vi "Parse Parameters File.vi"(8 "error in":errorcluster, 11 "path to XML document":path caption="path to parameters xml") -> (0 "error out":errorcluster, 2 "board configuration out":T1 {"portConfiguration"."Rx_UDP"."Tx_UDP"."FilterMode" items=["FDX_RX_VL_FLT_DIS", "FDX_RX_VL_FLT_ENA ", "FDX_RX_VL_FLT_ENA_INV"]; "portConfiguration"."Rx_UDP"."Tx_UDP"."VLBufSize" format="%.0x"; "portConfiguration"."Rx_UDP"."Tx_UDP"."VerificationMode" items=["FDX_RX_VL_CHECK_ENA_DEFAULT"=65535, "FDX_RX_VL_CHECK_REDMAM"=16, "DX_RX_VL_CHECK_TRAFIC"=8, "FDX_RX_VL_CHECK_FRAMESIZE"=4, "FDX_RX_VL_CHECK_SNINTEG"=2, "FDX_RX_VL_CHECK_INVPAC"=1, "FDX_RX_VL_CHECK_DISA"=0]; "portConfiguration"."Tx_UDP"."tx_udp_setup"."interfaceID" format="%.0b"; "portConfiguration"."Tx_UDP"."tx_udp_setup"."NetSelect" items=["FDX_TX_FRAME_DLY_A"=0, "FDX_TX_FRAME_DLY_B"=1, "FDX_TX_FRAME_BOTH "=3, "FDX_TX_FRAME_ONLY_A"=4, "FDX_TX_FRAME_ONLY_B "=5]; "portConfiguration"."Rx_Monitor"."Strobe" items=["FDX_MON_STROBE_DIS", "FDX_MON_STROBE_STOP", "FDX_MON_STROBE_START"]; "portConfiguration"."Rx_Monitor"."CaptureMode" items=["FDX_MON_SINGLE ", "FDX_MON_CONTINUOUS", "FDX_MON_SELECTIVE", "FDX_MON_RECORDING", "FDX_MON_REROS", "FDX_MON_HMU"]; "portConfiguration"."Rx_Monitor"."DefaultCronoMode" items=["FDX_RX_DEFAULT_ENA_CNT", "FDX_RX_DEFAULT_MON_ENA_ALL", "FDX_RX_DEFAULT_MON_ENA_GOOD"]; "portConfiguration"."Tx_Generic"."Frame Headers"."Frame header"."PhysErrorInjection" items=["FDX_TX_FRAME_ERR_OFF", "FDX_TX_FRAME_ERR_CRC", "FDX_TX_FRAME_ERR_ALI", "FDX_TX_FRAME_ERR_PRE", "FDX_TX_FRAME_ERR_PHY"]; "portConfiguration"."Tx_Generic"."Frame Headers"."Frame header"."PayloadGenerationMode" items=["FDX_TX_FRAME_PGM_USER", "FDX_TX_FRAME_PGM_IP_PART", "FDX_TX_FRAME_PGM_IP_PART_TT", "FDX_TX_FRAME_PGM_IP_FULL", "FDX_TX_FRAME_PGM_IP_FULL_TT"]; "portConfiguration"."Tx_Generic"."Frame Headers"."Frame header"."PayloadBufferMode" items=["FDX_TX_FRAME_PBM_STD", "FDX_TX_FRAME_PBM_MAC", "FDX_TX_FRAME_PBM_UDP", "FDX_TX_FRAME_PBM_FULL"]; "portConfiguration"."Tx_Generic"."Frame Headers"."Frame header"."NetSelect" items=["FDX_TX_FRAME_DLY_A"=0, "FDX_TX_FRAME_DLY_B"=1, "FDX_TX_FRAME_BOTH "=3, "FDX_TX_FRAME_ONLY_A"=4, "FDX_TX_FRAME_ONLY_B "=5]; "portConfiguration"."Tx_Generic"."Frame Headers"."Frame header"."FrameStartMode" items=["FDX_TX_FRAME_START_IFG", "FDX_TX_FRAME_START_PGWT", "FDX_TX_FRAME_START_TRG", "FDX_TX_FRAME_START_TRG_D"]; "portConfiguration"."Tx_Generic"."tx_generic_setup"."StartMode" items=["FDX_STOP", "FDX_START", "FDX_START_TRG", "FDX_START_TIME"]; "boardSetup"."portConfig" items=["FDX_SINGLE", "FDX_REDUNDANT"]; "boardSetup"."portSpeed" items=["FDX_100MBIT", "FDX_10MBIT", "FDX_AUTO_100MBIT", "FDX_AUTO_10MBIT", "FDX_AUTO_ERROR", "FDX_1000MBIT"]}, 3 "path to XML document out":path caption="path to parameters xml")   [LabVIEW 2020, in "AIM ARINC 664 Import.lvlib"]
uses:
  AIM ARINC 664 Import.lvlib
  <vilib>/xml/NI_XML.lvlib
  <resource>/objmgr/DOMUserDefRef.rc
  _typedefs/Board Top Level Configuration.ctl
  _typedefs/board_setup.ctl
  _typedefs/port_tx_udp_sap.ctl
  _typedefs/port_tx_udp_comm.ctl
  _typedefs/tx_udp_setup.ctl
  _typedefs/port_setup.ctl
  _typedefs/port_configuration.ctl
  _typedefs/port_rx_udp_sap.ctl
  _typedefs/port_rx_udp_comm.ctl
  _typedefs/rx_udp_setup.ctl
  _typedefs/frame_parameter.ctl
  _typedefs/frame_parameter_definition.ctl
  _typedefs/session_tx_generic.ctl
  _typedefs/frame_tx_generic_seqNumberOffset.ctl
  _typedefs/frame_tx_generic_seqNumberInit.ctl
  _typedefs/tx_generic_setup.ctl
  _typedefs/session_rx_monitor.ctl
  <vilib>/xml/Load XML File.vi
  _typedefs/frame_tx_generic.ctl
  Shared/Encoding (Arinc664).ctl
panel:
  out "parse errors":string
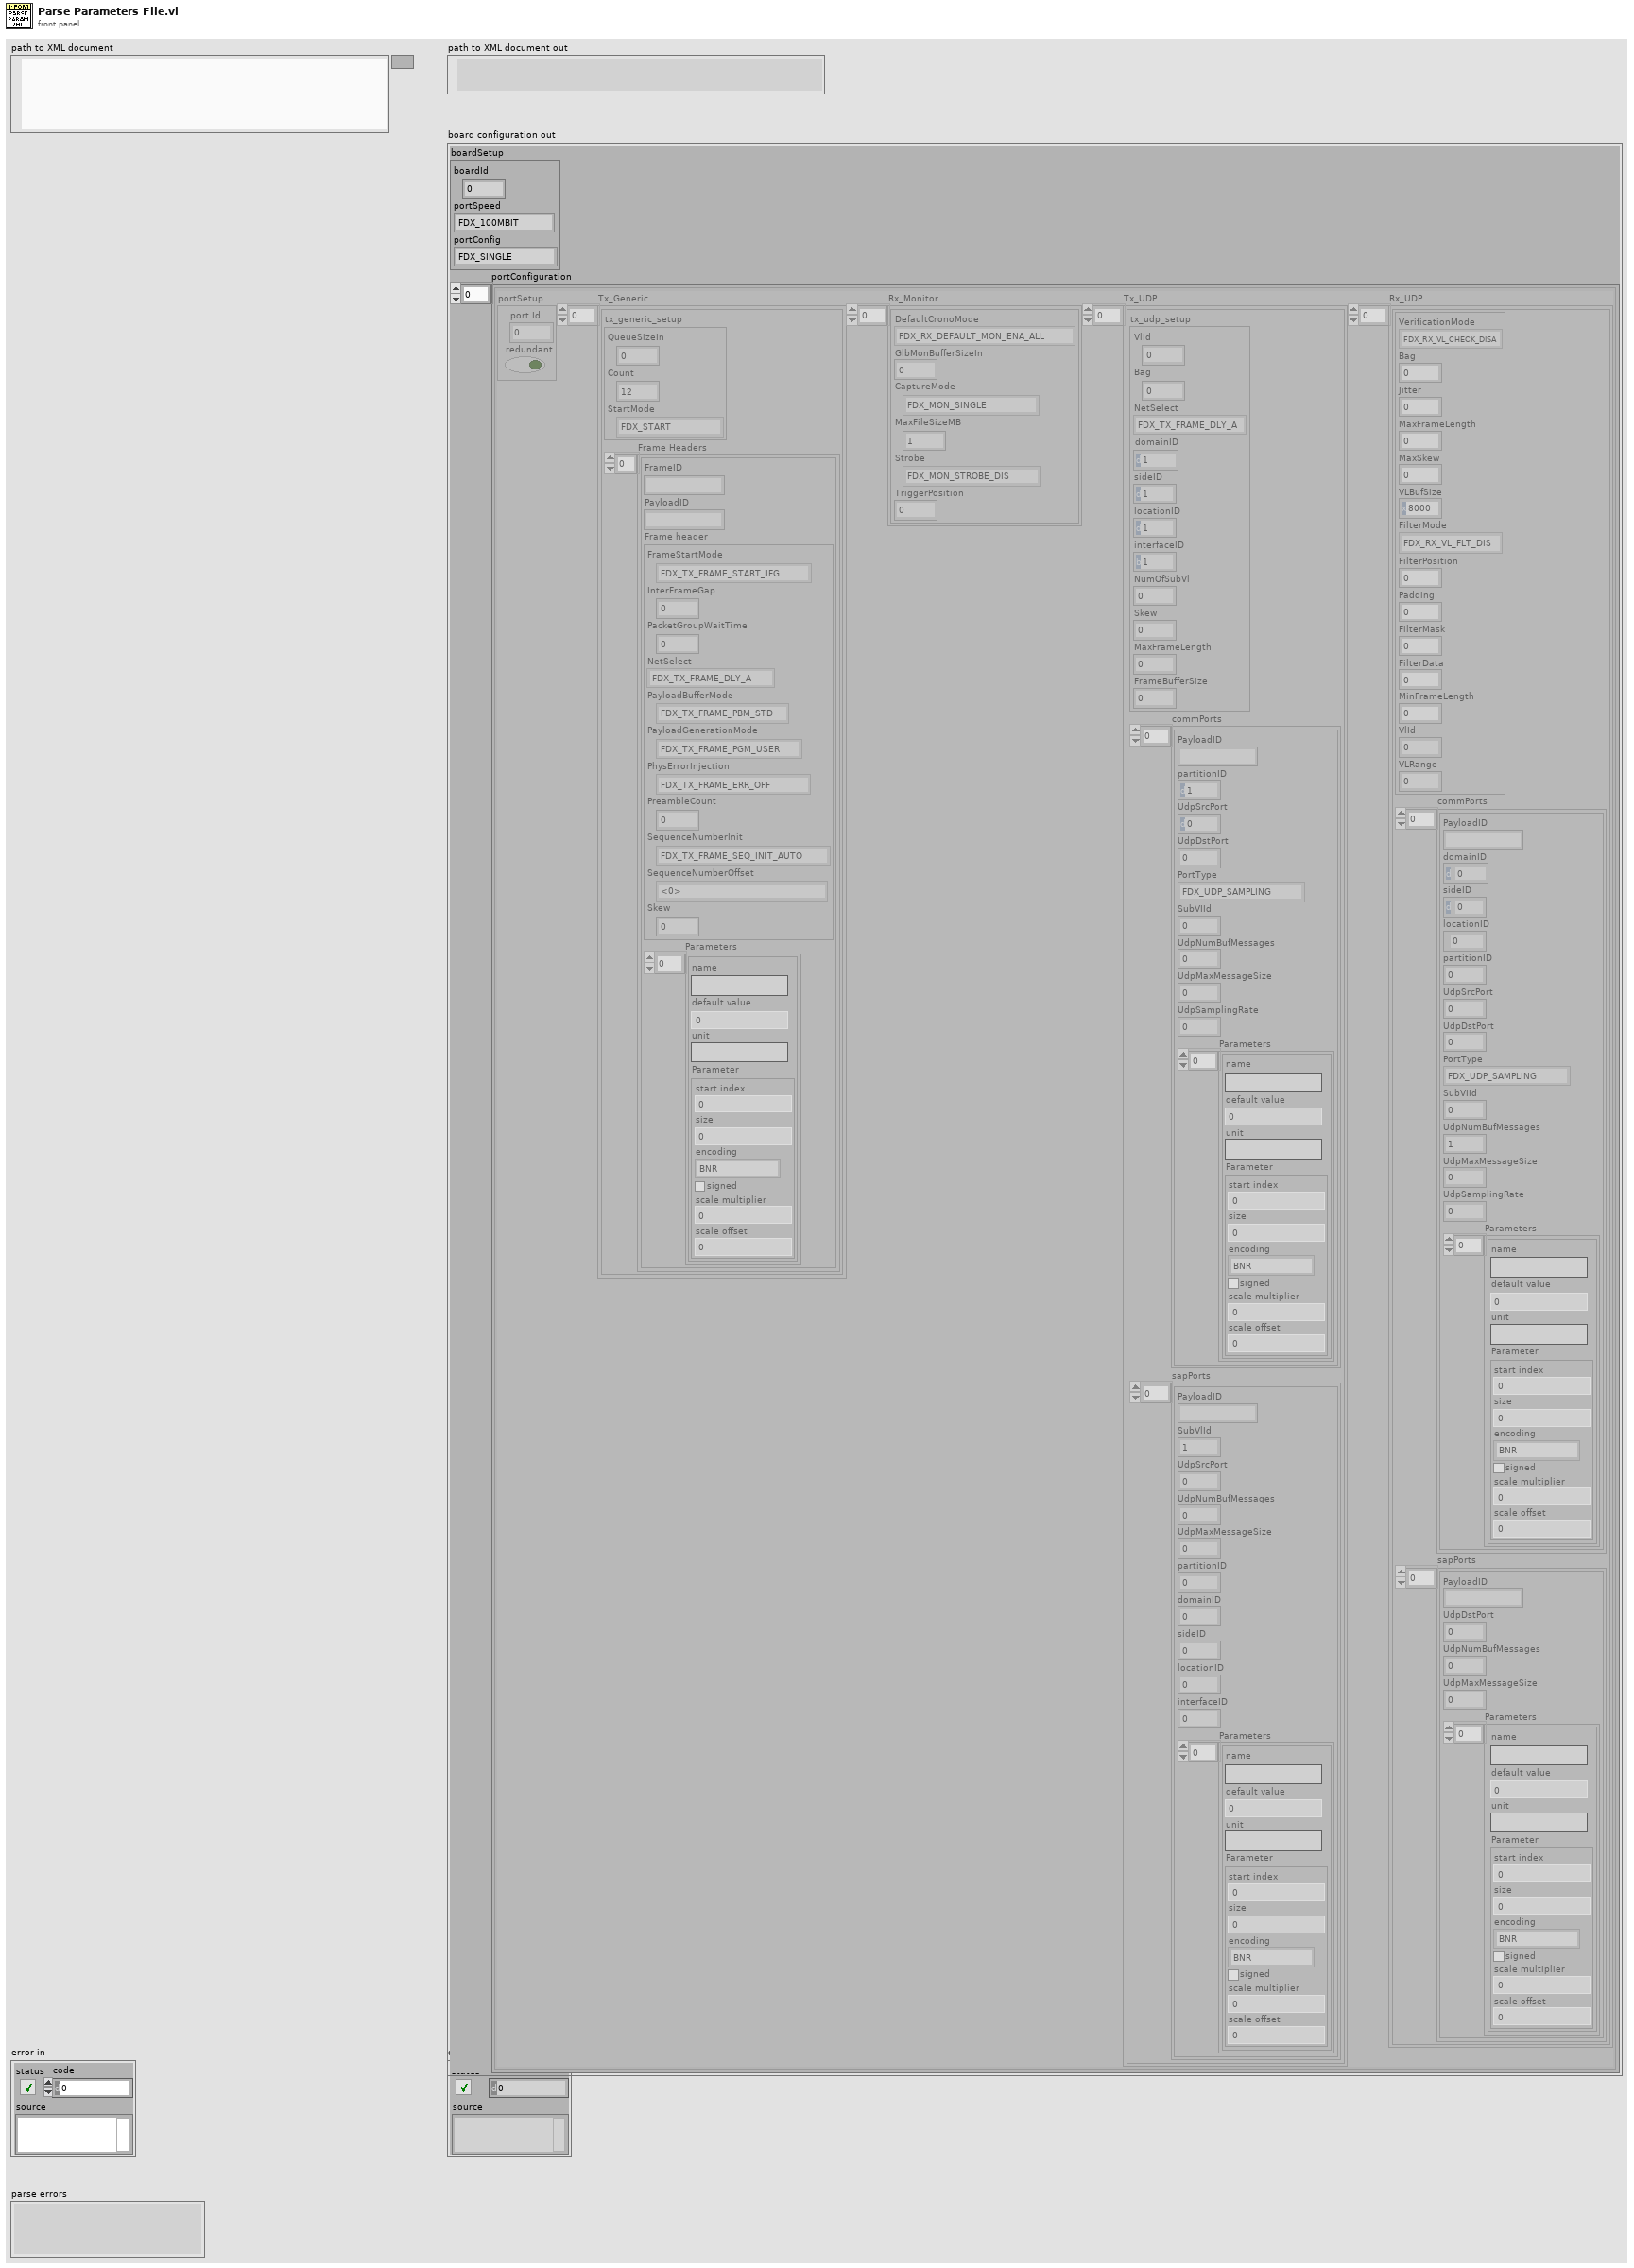
[diagram p1: front panel]
types:
  T1 = typedef "AIM ARINC 664 Import.lvlib/Board Top Level Configuration.ctl" = cluster{"boardSetup":T2, "portConfiguration":T3[]}
  T2 = typedef "AIM ARINC 664 Import.lvlib/board_setup.ctl" = cluster{"boardId":u32, "portSpeed":u32, "portConfig":u32}
  T3 = typedef "AIM ARINC 664 Import.lvlib/port_configuration.ctl" = cluster{"portSetup":T4, "Tx_Generic":T5[], "Rx_Monitor":cluster{"DefaultCronoMode":u32, "GlbMonBufferSizeIn":u32, "CaptureMode":u32, "MaxFileSizeMB":u32, "Strobe":u32, "TriggerPosition":u32}[], "Tx_UDP":cluster{"tx_udp_setup":cluster{"VlId":i32, "Bag":i32, "NetSelect":u32, "domainID":u8, "sideID":u8, "locationID":u8, "interfaceID":u8, "NumOfSubVl":u16, "Skew":u32, "MaxFrameLength":u32, "FrameBufferSize":u32}, "commPorts":T13[], "sapPorts":T14[]}[], "Rx_UDP":cluster{"Tx_UDP":T15, "commPorts":T16[], "sapPorts":T17[]}[]}
  T4 = typedef "AIM ARINC 664 Import.lvlib/port_setup.ctl" = cluster{"port Id":u32, "redundant":bool}
  T5 = typedef "AIM ARINC 664 Import.lvlib/session_tx_generic.ctl" = cluster{"tx_generic_setup":T6, "Frame Headers":T7[]}
  T6 = typedef "AIM ARINC 664 Import.lvlib/tx_generic_setup.ctl" = cluster{"QueueSizeIn":u32, "Count":i32, "StartMode":i32}
  T7 = typedef "AIM ARINC 664 Import.lvlib/frame_tx_generic.ctl" = cluster{"FrameID":string, "PayloadID":string, "Frame header":cluster{"FrameStartMode":i32, "InterFrameGap":i32, "PacketGroupWaitTime":i32, "NetSelect":u32, "PayloadBufferMode":i32, "PayloadGenerationMode":i32, "PhysErrorInjection":i32, "PreambleCount":i32, "SequenceNumberInit":T8, "SequenceNumberOffset":T9, "Skew":i32}, "Parameters":T10[]}
  T8 = typedef "AIM ARINC 664 Import.lvlib/frame_tx_generic_seqNumberInit.ctl" = i32
  T9 = typedef "AIM ARINC 664 Import.lvlib/frame_tx_generic_seqNumberOffset.ctl" = i32
  T10 = typedef "AIM ARINC 664 Import.lvlib/frame_parameter.ctl" = cluster{"name":string, "default value":dbl, "unit":string, "Parameter":T11}
  T11 = typedef "AIM ARINC 664 Import.lvlib/frame_parameter_definition.ctl" = cluster{"start index":i32, "size":i32, "encoding":T12, "signed":bool, "scale multiplier":dbl, "scale offset":dbl}
  T12 = typedef "Encoding (Arinc664).ctl" = u16
  T13 = typedef "AIM ARINC 664 Import.lvlib/port_tx_udp_comm.ctl" = cluster{"PayloadID":string, "partitionID":u8, "UdpSrcPort":u16, "UdpDstPort":u16, "PortType":enum16{"FDX_UDP_SAMPLING", "FDX_UDP_QUEUING"}, "SubVIId":u32, "UdpNumBufMessages":u32, "UdpMaxMessageSize":u32, "UdpSamplingRate":u32, "Parameters":T10[]}
  T14 = typedef "AIM ARINC 664 Import.lvlib/port_tx_udp_sap.ctl" = cluster{"PayloadID":string, "SubVlId":u8, "UdpSrcPort":u16, "UdpNumBufMessages":u32, "UdpMaxMessageSize":u32, "partitionID":u8, "domainID":u8, "sideID":u8, "locationID":u8, "interfaceID":u8, "Parameters":T10[]}
  T15 = typedef "AIM ARINC 664 Import.lvlib/rx_udp_setup.ctl" = cluster{"VerificationMode":u32, "Bag":u32, "Jitter":u32, "MaxFrameLength":u32, "MaxSkew":u32, "VLBufSize":u32, "FilterMode":u32, "FilterPosition":u32, "Padding":u32, "FilterMask":u32, "FilterData":u32, "MinFrameLength":u32, "VlId":u16, "VLRange":u32}
  T16 = typedef "AIM ARINC 664 Import.lvlib/port_rx_udp_comm.ctl" = cluster{"PayloadID":string, "domainID":u8, "sideID":u8, "locationID":u8, "partitionID":u8, "UdpSrcPort":u16, "UdpDstPort":u16, "PortType":enum16{"FDX_UDP_SAMPLING", "FDX_UDP_QUEUING"}, "SubVIId":u32, "UdpNumBufMessages":u32, "UdpMaxMessageSize":u32, "UdpSamplingRate":u32, "Parameters":T10[]}
  T17 = typedef "AIM ARINC 664 Import.lvlib/port_rx_udp_sap.ctl" = cluster{"PayloadID":string, "UdpDstPort":u16, "UdpNumBufMessages":u32, "UdpMaxMessageSize":u32, "Parameters":T10[]}
  T18 = typedef "AIM ARINC 664 Import.lvlib/session_rx_monitor.ctl" = cluster{"DefaultCronoMode":u32, "GlbMonBufferSizeIn":u32, "CaptureMode":u32, "MaxFileSizeMB":u32, "Strobe":u32, "TriggerPosition":u32}
  T19 = cluster{"rx_udp_setup":T15, "commPorts":T16[], "sapPorts":T17[]}[]
  T20 = typedef "AIM ARINC 664 Import.lvlib/tx_udp_setup.ctl" = cluster{"VlId":i32, "Bag":i32, "NetSelect":u32, "domainID":u8, "sideID":u8, "locationID":u8, "interfaceID":u8, "NumOfSubVl":u16, "Skew":u32, "MaxFrameLength":u32, "FrameBufferSize":u32}
  T21 = cluster{"tx_udp_setup":T20, "commPorts":T13[], "sapPorts":T14[]}[]
  T22 = cluster{"tx_udp_setup":T20, "commPorts":T13[], "sapPorts":T14[]}
  T23 = cluster{"rx_udp_setup":T15, "commPorts":T16[], "sapPorts":T17[]}
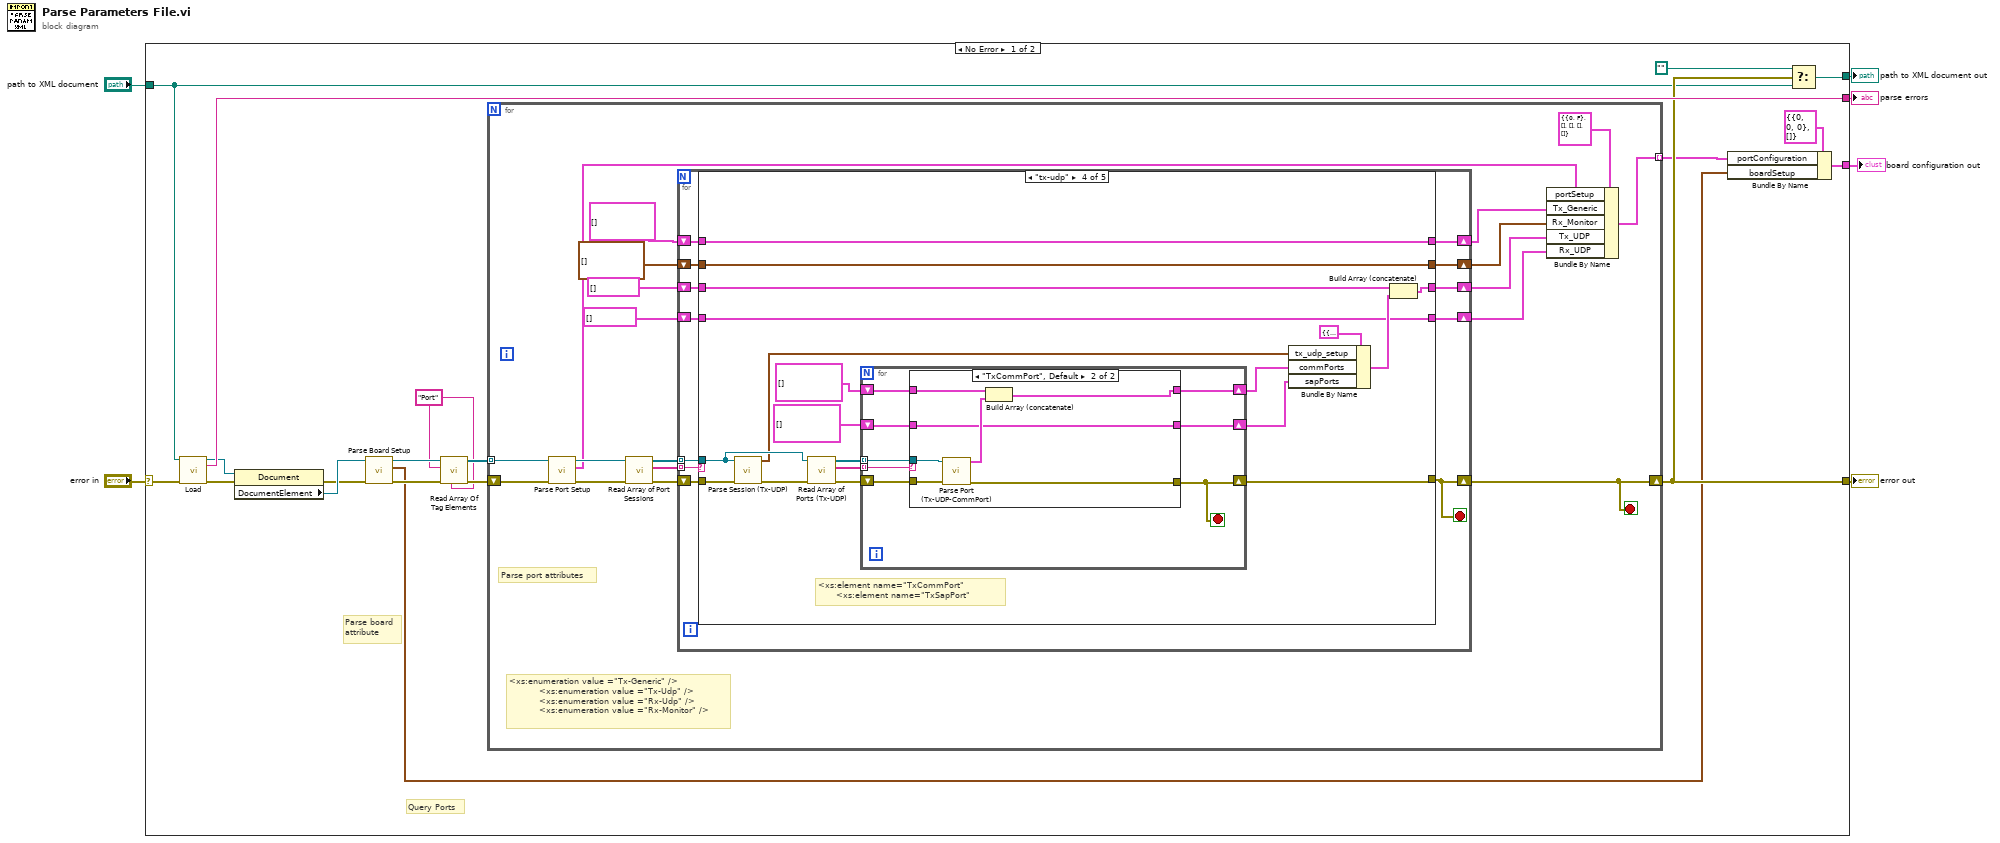
[diagram p0: block diagram]
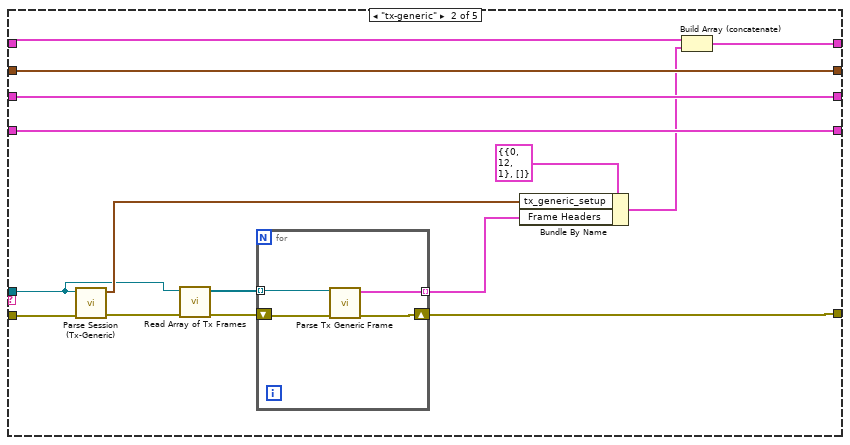
[diagram p3: hidden frame]
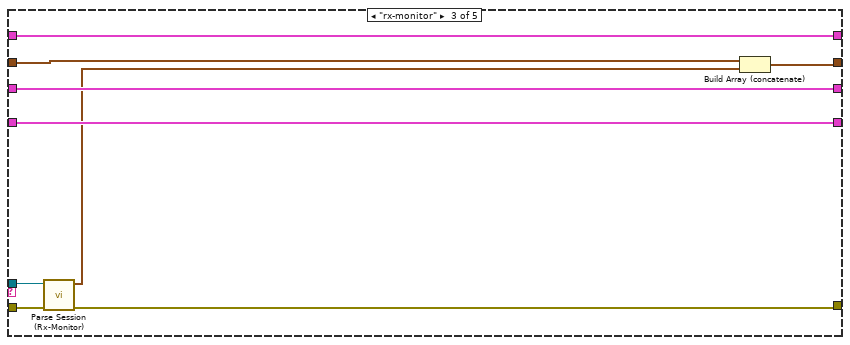
[diagram p4: hidden frame]
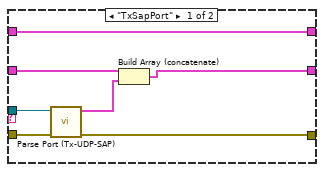
[diagram p5: hidden frame]
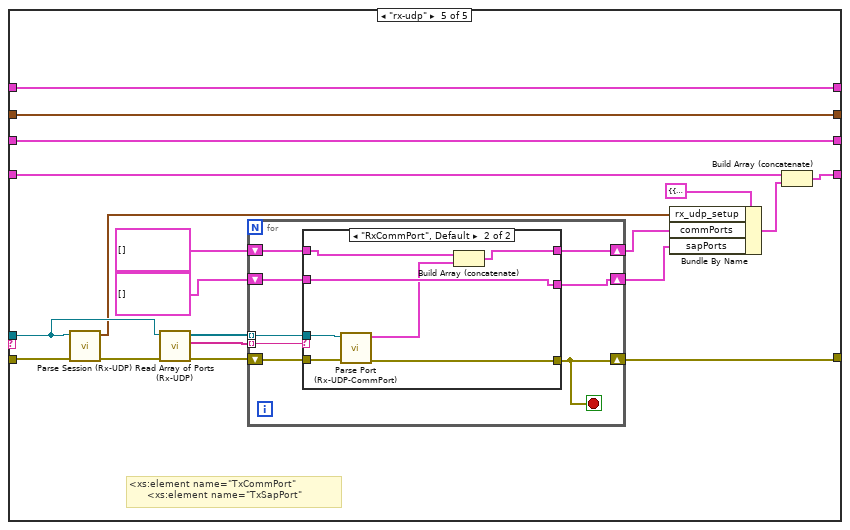
[diagram p6: hidden frame]
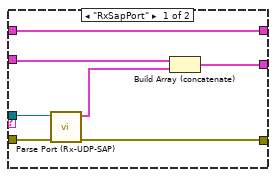
[diagram p7: hidden frame]
diagram:
  n1 = case shown="No Error" "error in" {
    selector: "error in" -> [w20 w172]
    tunnel: [w25 _] -> w6
    tunnel: [w19 w172] -> w5
    tunnel: "path to XML document" -> [w17 _]
    tunnel: [w18 _] -> w2
    tunnel: [w10 _] -> w1
    frame No Error {
      w8 = "Port" ("Tag Name")
      # "Query Ports"
      # "Parse board\nattribute"
      n2 = call-poly <vilib>:"Load.vi"("path to XML document"=w17, "error in (no error)"=w20) -> ("DOM document out"=w24:refnum<k20>, "parse errors"=w25:string, "error out"=w23:errorcluster)  [unwired: 11 in]
      n3 = property class="Document"(reference=w24, error in=w23) -> (error out=w13:errorcluster, "DocumentElement"=w14:refnum<k20>)  [unwired: 1 out]
      n4 = call "Parse Board Setup.vi"("error in"=w13, "node in"=w14) -> ("error out"=w12:errorcluster, "portSetup"=w7:T2, "node out"=w11:refnum<k20>)  [unwired: 7 in]
      n5 = call "Read Array Of Tag Elements.vi"("error text in"=w8, "error in"=w12, "tag name"=w8, "node in"=w11) -> ("error out"=w22:errorcluster, "array of elements"=w21:refnum<k20>[])  [unwired: 6 in]
      n6 = for {
        tunnel: w21 -> [w40] mode=indexing
        shift-right: [w41] -> w19
        shift-left: w22 -> [w39]
        tunnel: [w35] -> w9 mode=indexing
        stop <- w41 stop-if-true
        # "<xs:enumeration value =\"Tx-Generic\" />\n          <xs:enumeration value =\"Tx-Udp\" />\n          <xs:enumeration value =\"Rx-Udp\" />\n          <xs:enumeration value =\"Rx-Monitor\" />"
        # "Parse port attributes"
        n7 = call "Parse Port Setup.vi"("error in"=w39, "node in"=w40) -> ("error out"=w38:errorcluster, "portSetup"=w34:T4, "node out"=w37:refnum<k20>)  [unwired: 7 in]
        n8 = call "Read Array of Port Sessions.vi"("error in"=w38, "port node in"=w37) -> ("error out"=w43:errorcluster, "session type"=w44:string[], "port node out"=w42:refnum<k20>[])  [unwired: 7 in]
        n9 = for {
          tunnel: w44 -> [w56] mode=indexing
          tunnel: w42 -> [w54] mode=indexing
          shift-right: [w53] -> w41
          shift-left: w43 -> [w55]
          shift-right: [w49] -> w28
          shift-left: T5[] [] ("Array") -> [w50]
          shift-right: [w45] -> w32
          shift-left: T18[] [] ("Array") -> [w51]
          shift-right: [w48] -> w31
          shift-left: T21 [] ("Tx_UDP") -> [w52]
          shift-right: [w46] -> w29
          shift-left: T19 [] ("Rx_UDP") -> [w47]
          stop <- w53 stop-if-true
          n10 = case shown="\"tx-udp\"" w56 {
            tunnel: w55 -> [w61 w76 w88 w101 w139]
            tunnel: w54 -> [_ w71 w89 w99 w137]
            tunnel: [w61 w67 w87 w105 w149] -> w53
            tunnel: w52 -> [w59 w75 w85 w103 w144]
            tunnel: w51 -> [w57 w65 w81 w90 w131]
            tunnel: w50 -> [w60 w63 w86 w104 w145]
            tunnel: [w60 w62 w86 w104 w145] -> w49
            tunnel: [w59 w75 w85 w98 w144] -> w48
            tunnel: w47 -> [w58 w74 w84 w92 w143]
            tunnel: [w58 w74 w84 w92 w141] -> w46
            tunnel: [w57 w65 w82 w90 w131] -> w45
            frame Default {
            }
            frame "tx-generic" {
              n11 = call "Parse Session (Tx-Generic).vi"("error in"=w76, "node in"=w71) -> ("error out"=w70:errorcluster, "tx_generic_setup"=w72:T6)  [unwired: 8 in]
              n12 = call "Read Array of Tx Frames.vi"("error in"=w70, "port node in"=w71) -> ("error out"=w69:errorcluster, "te generic frames"=w68:refnum<k20>[])  [unwired: 8 in]
              n13 = for {
                tunnel: w68 -> [w78] mode=indexing
                shift-right: [w77] -> w67
                shift-left: w69 -> [w79]
                tunnel: [w80] -> w66 mode=indexing
                n14 = call "Parse Tx Generic Frame.vi"("error in"=w79, "node in"=w78) -> ("error out"=w77:errorcluster, "Frame Generic"=w80:T7)  [unwired: 8 in]
              }
              n15 = Bundle By Name(cluster=T5 {"tx_generic_setup"={"QueueSizeIn"=0, "Count"=12, "StartMode"=1}, "Frame Headers"=[]} ("session_tx_generic"), "tx_generic_setup"=w72, "Frame Headers"=w66) -> (w64:T5)
              n16 = Build Array (concatenate)(w63, w64) -> (w62:T5[])
            }
            frame "rx-monitor" {
              n17 = call "Parse Session (Rx-Monitor).vi"("error in"=w88, "node in"=w89) -> ("error out"=w87:errorcluster, "session_rx_monitor"=w83:T18)  [unwired: 8 in]
              n18 = Build Array (concatenate)(w81, w83) -> (w82:T18[])
            }
            frame "tx-udp" {
              # "<xs:element name=\"TxCommPort\" \n      <xs:element name=\"TxSapPort\""
              n19 = call "Parse Session (Tx-UDP).vi"("error in"=w101, "node in"=w99) -> ("error out"=w100:errorcluster, "tx udp session out"=w91:T20)  [unwired: 8 in]
              n20 = call "Read Array of Ports (Tx-UDP).vi"("error in"=w100, "port node in"=w99) -> ("error out"=w108:errorcluster, "txudp ports types"=w107:string[], "tx udp port nodes"=w106:refnum<k20>[])  [unwired: 7 in]
              n21 = for {
                tunnel: w107 -> [w116] mode=indexing
                tunnel: w106 -> [w114] mode=indexing
                shift-right: [w113] -> w105
                shift-left: w108 -> [w115]
                shift-right: [w111] -> w94
                shift-left: T13[] [] ("commPorts") -> [w112]
                shift-right: [w109] -> w93
                shift-left: T14[] [] ("sapPorts") -> [w110]
                stop <- w113 stop-if-true
                n22 = case shown="\"TxCommPort\", Default" w116 {
                  tunnel: w115 -> [w122 w129]
                  tunnel: w114 -> [w123 w130]
                  tunnel: [w117 w128] -> w113
                  tunnel: w112 -> [w121 w127]
                  tunnel: [w121 w124] -> w111
                  tunnel: w110 -> [w120 w125]
                  tunnel: [w118 w125] -> w109
                  frame "TxSapPort" {
                    n23 = call "Parse Port (Tx-UDP-SAP).vi"("error in"=w122, "node in"=w123) -> ("error out"=w117:errorcluster, "tx udp sap port out"=w119:T14)  [unwired: 8 in]
                    n24 = Build Array (concatenate)(w120, w119) -> (w118:T14[])
                  }
                  frame "TxCommPort", Default {
                    n25 = call "Parse Port (Tx-UDP-CommPort).vi"("error in"=w129, "node in"=w130) -> ("error out"=w128:errorcluster, "tx udp comm port out"=w126:T13)  [unwired: 8 in]
                    n26 = Build Array (concatenate)(w127, w126) -> (w124:T13[])
                  }
                }
              }
              n27 = Bundle By Name(cluster=T22 {"tx_udp_setup"={"VlId"=0, "Bag"=0, "NetSelect"=0, "domainID"=0, "sideID"=0, "locationID"=0, "interfaceID"=0, "NumOfSubVl"=0, "Skew"=0, "MaxFrameLength"=0, "FrameBufferSize"=0}, "commPorts"=[], "sapPorts"=[]} ("Tx_UDP"), "tx_udp_setup"=w91, "commPorts"=w94, "sapPorts"=w93) -> (w97:T22)
              n28 = Build Array (concatenate)(w103, w97) -> (w98:T21)
            }
            frame "rx-udp" {
              # "<xs:element name=\"TxCommPort\" \n      <xs:element name=\"TxSapPort\""
              n29 = call "Parse Session (Rx-UDP).vi"("error in"=w139, "node in"=w137) -> ("error out"=w138:errorcluster, "tx udp session out"=w136:T15)  [unwired: 8 in]
              n30 = call "Read Array of Ports (Rx-UDP).vi"("error in"=w138, "port node in"=w137) -> ("error out"=w146:errorcluster, "rx udp ports types"=w147:string[], "rx udp port nodes"=w148:refnum<k20>[])  [unwired: 7 in]
              n31 = for {
                tunnel: w147 -> [w157] mode=indexing
                tunnel: w148 -> [w155] mode=indexing
                shift-right: [w154] -> w149
                shift-left: w146 -> [w156]
                shift-right: [w150] -> w133
                shift-left: T16[] [] ("commPorts") -> [w153]
                shift-right: [w151] -> w132
                shift-left: T17[] [] ("sapPorts") -> [w152]
                stop <- w154 stop-if-true
                n32 = case shown="\"RxCommPort\", Default" w157 {
                  tunnel: w156 -> [w163 w170]
                  tunnel: w155 -> [w164 w171]
                  tunnel: [w162 w169] -> w154
                  tunnel: w153 -> [w158 w167]
                  tunnel: w152 -> [w160 w168]
                  tunnel: [w159 w168] -> w151
                  tunnel: [w158 w165] -> w150
                  frame "RxSapPort" {
                    n33 = call "Parse Port (Rx-UDP-SAP).vi"("error in"=w163, "node in"=w164) -> ("error out"=w162:errorcluster, "rx udp sap port out"=w161:T17)  [unwired: 8 in]
                    n34 = Build Array (concatenate)(w160, w161) -> (w159:T17[])
                  }
                  frame "RxCommPort", Default {
                    n35 = call "Parse Port (Rx-UDP-CommPort).vi"("error in"=w170, "node in"=w171) -> ("error out"=w169:errorcluster, "rx udp comm port out"=w166:T16)  [unwired: 8 in]
                    n36 = Build Array (concatenate)(w167, w166) -> (w165:T16[])
                  }
                }
              }
              n37 = Bundle By Name(cluster=T23 {"rx_udp_setup"={"VerificationMode"=0, "Bag"=0, "Jitter"=0, "MaxFrameLength"=0, "MaxSkew"=0, "VLBufSize"=0, "FilterMode"=0, "FilterPosition"=0, "Padding"=0, "FilterMask"=0, "FilterData"=0, "MinFrameLength"=0, "VlId"=0, "VLRange"=0}, "commPorts"=[], "sapPorts"=[]} ("Tx_UDP"), "rx_udp_setup"=w136, "commPorts"=w133, "sapPorts"=w132) -> (w140:T23)
              n38 = Build Array (concatenate)(w143, w140) -> (w141:T19)
            }
          }
        }
        n39 = Bundle By Name(cluster=T3 {"portSetup"={"port Id"=0, "redundant"=FALSE}, "Tx_Generic"=[], "Rx_Monitor"=[], "Tx_UDP"=[], "Rx_UDP"=[]} ("portConfiguration"), "portSetup"=w34, "Tx_Generic"=w28, "Rx_Monitor"=w32, "Tx_UDP"=w31, "Rx_UDP"=w29) -> (w35:T3)
      }
      n40 = Bundle By Name(cluster=T1 {"boardSetup"={"boardId"=0, "portSpeed"=0, "portConfig"=0}, "portConfiguration"=[]}, "portConfiguration"=w9, "boardSetup"=w7) -> (w10:T1)
      n41 = Select(t=path "", s=w19, f=w17) -> (s? t:f=w18:path)
    }
    frame Error {
    }
  }
  "parse errors" <- w6
  "error out" <- w5
  "path to XML document out" <- w2
  "board configuration out" <- w1
